vi "Stage Monitor.vi"() -> ()   [LabVIEW 2014]
uses:
  Controls/StageStates.ctl
panel:
  in  "P541 Only":bool
  in  "Monitoring":bool
  in  "Exit":bool
  out "Monitor 5":cluster{"Numeric":dbl}(graph) caption="N664"
  out "Monitor 4":cluster{"Numeric":dbl, "Numeric":dbl}(graph) caption="N664"
  out "Monitor 3":T1(graph) caption="N664"
  out "Monitor 2":T1(graph) caption="N664"
  out "Monitor 1":cluster{"Numeric":dbl}(graph) caption="N664"
  in  "Stages":T2
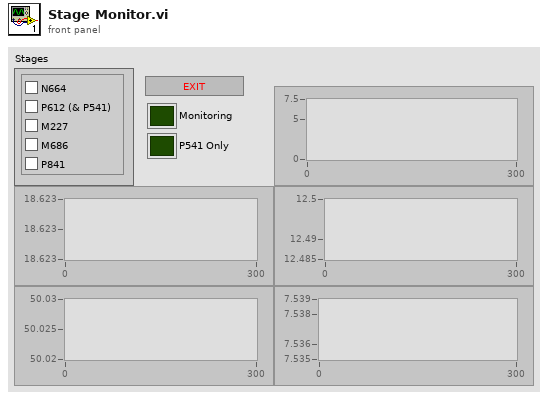
[diagram p1: front panel]
types:
  T1 = cluster{"Numeric":dbl, "Numeric":dbl, "Numeric":dbl}
  T2 = cluster{"N664":bool, "P612":bool, "M227":bool, "M686":bool, "P841":bool}
  T3 = enum8{"Enabled", "Disabled", "Disabled and Grayed Out"}
  T4 = typedef "StageStates.ctl" = enum16{"POSITION", "MVR", "MOVE", "HALT", "ONTARGET", "ERROR", "EXIT", "HOME", "ZEROPOS", "NANOPOS", "QUIT", "ANALOG"}
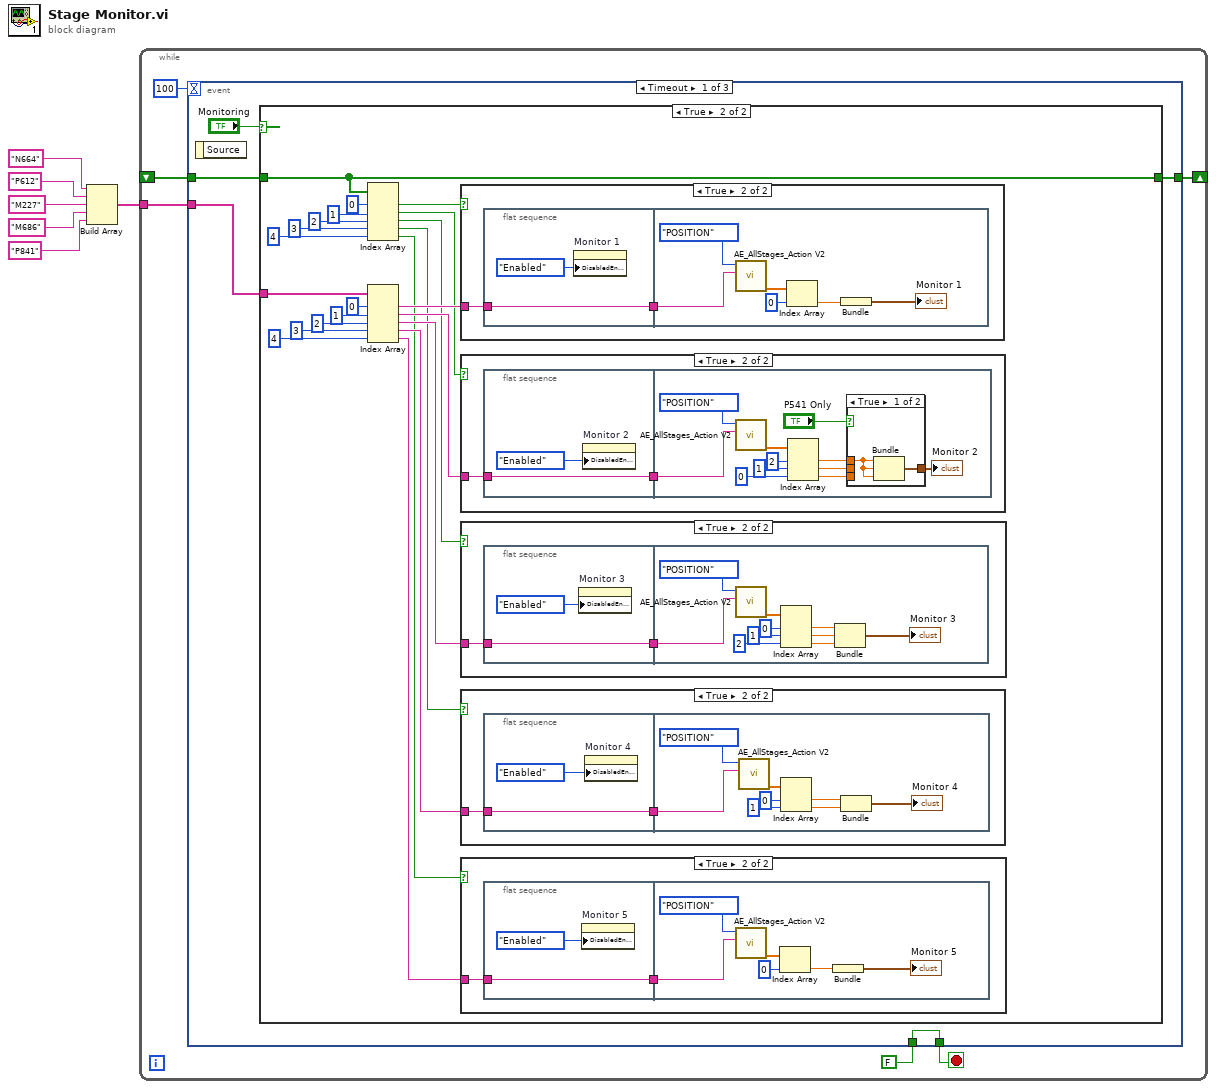
[diagram p0: block diagram]
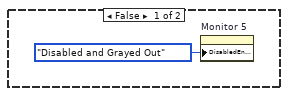
[diagram p3: hidden frame]
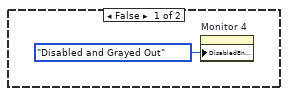
[diagram p4: hidden frame]
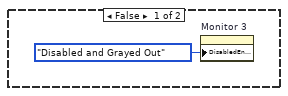
[diagram p5: hidden frame]
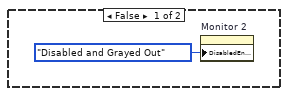
[diagram p6: hidden frame]
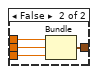
[diagram p7: hidden frame]
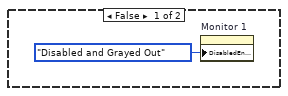
[diagram p8: hidden frame]
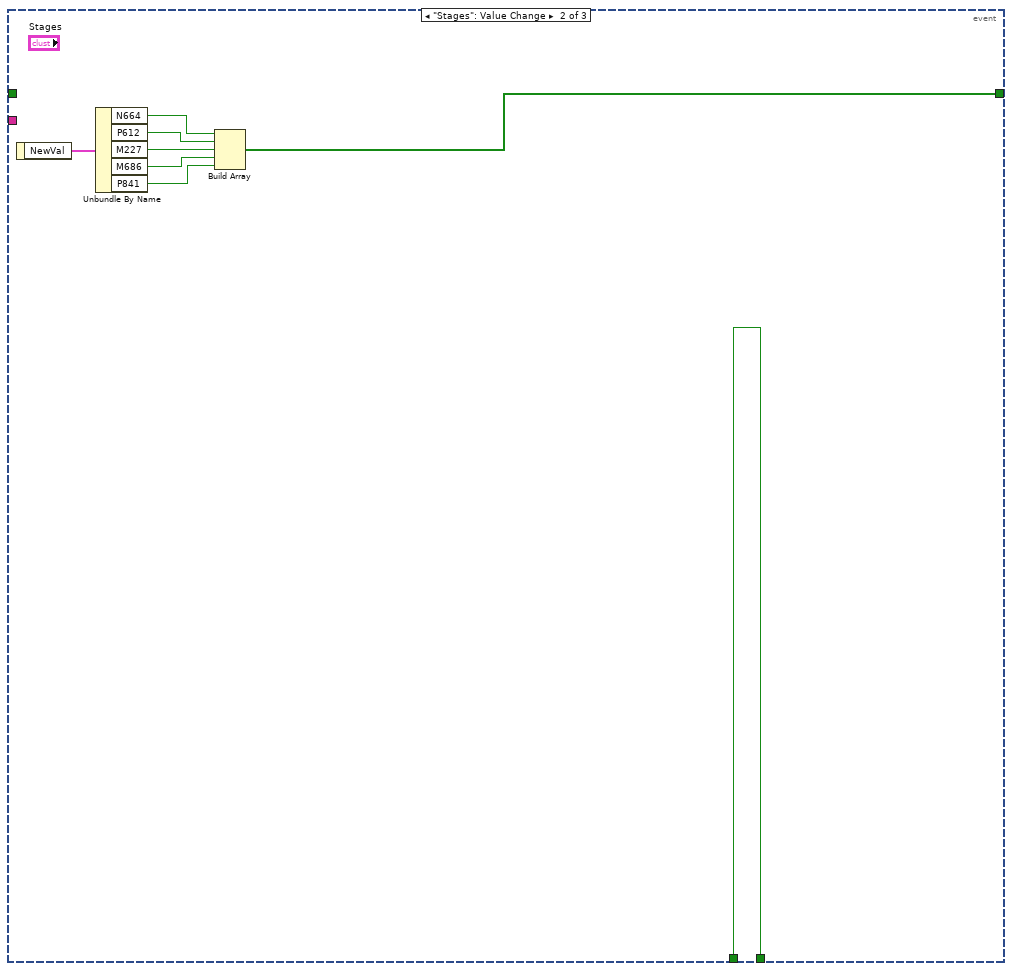
[diagram p9: hidden frame]
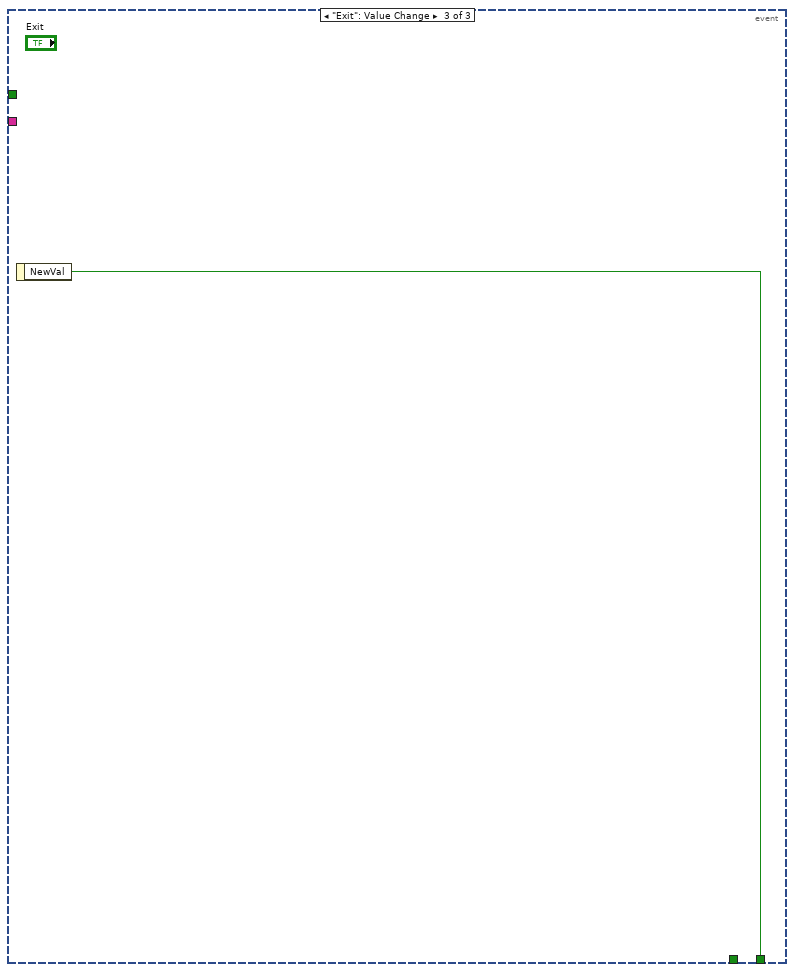
[diagram p10: hidden frame]
diagram:
  n1 = Build Array("N664", "P612", "M227", "M686", "P841") -> (w1:string[])
  n2 = while {
    shift-right: [w9] -> _
    shift-left: _ -> [w8]
    tunnel: w1 -> [w7]
    stop <- w10 stop-if-true
    n3 = event shown="[0] Timeout" {
      selector: _ -> [_ _ _]
      dyn-events: _ -> [_ _ _]
      timeout: 100 -> [_ _ _]
      tunnel: FALSE -> [w17 w120 _]
      tunnel: [w17 w120 w121] -> w10
      tunnel: [w13 w113 _] -> w9
      tunnel: w8 -> [w15 _ _]
      tunnel: w7 -> [w14 _ _]
      event Timeout {
        n4 = event-data() -> ()  [unwired: 1 in, 1 out]
        n5 = case shown="True" "Monitoring" {
          tunnel: w15 -> [w18 w40]
          tunnel: w14 -> [_ w33]
          tunnel: [w18 w40] -> w13
          frame False {
          }
          frame True {
            n6 = Index Array(array=w40, index #1=0 ("index"), index #2=1 ("index"), index #3=2 ("index"), index #4=3 ("index"), index #5=4 ("index")) -> (element #1=w34:bool, element #2=w26:bool, element #3=w24:bool, element #4=w22:bool, element #5=w20:bool)
            n7 = Index Array(array=w33, index #1=0 ("index"), index #2=1 ("index"), index #3=2 ("index"), index #4=3 ("index"), index #5=4 ("index")) -> (element #1=w27:string, element #2=w25:string, element #3=w23:string, element #4=w21:string, element #5=w19:string)
            n8 = case shown="True" w34 {
              tunnel: w27 -> [_ w103]
              frame False {
                n9 = property on="Monitor 1" class="WFChart (strict)"("DisabledEnum"=T3."Disabled and Grayed Out" ("Disabled")) -> ()  [unwired: 2 in, 2 out]
              }
              frame True {
                n10 = flat-sequence {
                  tunnel: [w105] -> w104
                  tunnel: w103 -> [w105]
                  tunnel: w104 -> [w111]
                  frame #0 {
                    n11 = property on="Monitor 1" class="WFChart (strict)"("DisabledEnum"=T3."Enabled" ("Disabled")) -> ()  [unwired: 2 in, 2 out]
                  }
                  frame #1 {
                    n12 = call "AE_AllStages_Action V2.vi"("Stage ID"=w111, "Action"=StageStates."POSITION") -> ("Position Out"=w110:dbl[])  [unwired: 7 in, 2 out]
                    n13 = Index Array(array=w110, index=0) -> (element=w108:dbl)
                    n14 = Bundle("Numeric"=w108) -> (→"Monitor 1":cluster{"Numeric":dbl})  [unwired: 1 in]
                  }
                }
              }
            }
            n15 = case shown="True" w26 {
              tunnel: w25 -> [_ w81]
              frame False {
                n16 = property on="Monitor 2" class="WFChart (strict)"("DisabledEnum"=T3."Disabled and Grayed Out" ("Disabled")) -> ()  [unwired: 2 in, 2 out]
              }
              frame True {
                n17 = flat-sequence {
                  tunnel: [w83] -> w82
                  tunnel: w81 -> [w83]
                  tunnel: w82 -> [w94]
                  frame #0 {
                    n18 = property on="Monitor 2" class="WFChart (strict)"("DisabledEnum"=T3."Enabled" ("Disabled")) -> ()  [unwired: 2 in, 2 out]
                  }
                  frame #1 {
                    n19 = call "AE_AllStages_Action V2.vi"("Stage ID"=w94, "Action"=StageStates."POSITION") -> ("Position Out"=w93:dbl[])  [unwired: 7 in, 2 out]
                    n20 = Index Array(array=w93, index #1=2 ("index"), index #2=1 ("index"), index #3=0 ("index")) -> (element #1=w89:dbl, element #2=w88:dbl, element #3=w87:dbl)
                    n21 = case shown="True" "P541 Only" {
                      tunnel: w89 -> [w97 w101]
                      tunnel: w88 -> [_ w100]
                      tunnel: w87 -> [_ w99]
                      tunnel: [w96 w98] -> w85
                      frame True {
                        n22 = Bundle("Numeric"=w97, "Numeric"=w97, "Numeric"=w97) -> (w96:T1)  [unwired: 1 in]
                      }
                      frame False {
                        n23 = Bundle("Numeric"=w101, "Numeric"=w100, "Numeric"=w99) -> (w98:T1)  [unwired: 1 in]
                      }
                    }
                    "Monitor 2" <- w85
                  }
                }
              }
            }
            n24 = case shown="True" w24 {
              tunnel: w23 -> [_ w66]
              frame False {
                n25 = property on="Monitor 3" class="WFChart (strict)"("DisabledEnum"=T3."Disabled and Grayed Out" ("Disabled")) -> ()  [unwired: 2 in, 2 out]
              }
              frame True {
                n26 = flat-sequence {
                  tunnel: [w68] -> w67
                  tunnel: w66 -> [w68]
                  tunnel: w67 -> [w78]
                  frame #0 {
                    n27 = property on="Monitor 3" class="WFChart (strict)"("DisabledEnum"=T3."Enabled" ("Disabled")) -> ()  [unwired: 2 in, 2 out]
                  }
                  frame #1 {
                    n28 = call "AE_AllStages_Action V2.vi"("Stage ID"=w78, "Action"=StageStates."POSITION") -> ("Position Out"=w77:dbl[])  [unwired: 7 in, 2 out]
                    n29 = Index Array(array=w77, index #1=0 ("index"), index #2=1 ("index"), index #3=2 ("index")) -> (element #1=w73:dbl, element #2=w72:dbl, element #3=w71:dbl)
                    n30 = Bundle("Numeric"=w73, "Numeric"=w72, "Numeric"=w71) -> (→"Monitor 3":T1)  [unwired: 1 in]
                  }
                }
              }
            }
            n31 = case shown="True" w22 {
              tunnel: w21 -> [_ w53]
              frame False {
                n32 = property on="Monitor 4" class="WFChart (strict)"("DisabledEnum"=T3."Disabled and Grayed Out" ("Disabled")) -> ()  [unwired: 2 in, 2 out]
              }
              frame True {
                n33 = flat-sequence {
                  tunnel: [w55] -> w54
                  tunnel: w53 -> [w55]
                  tunnel: w54 -> [w63]
                  frame #0 {
                    n34 = property on="Monitor 4" class="WFChart (strict)"("DisabledEnum"=T3."Enabled" ("Disabled")) -> ()  [unwired: 2 in, 2 out]
                  }
                  frame #1 {
                    n35 = call "AE_AllStages_Action V2.vi"("Stage ID"=w63, "Action"=StageStates."POSITION") -> ("Position Out"=w62:dbl[])  [unwired: 7 in, 2 out]
                    n36 = Index Array(array=w62, index #1=0 ("index"), index #2=1 ("index")) -> (element #1=w59:dbl, element #2=w58:dbl)
                    n37 = Bundle("Numeric"=w59, "Numeric"=w58) -> (→"Monitor 4":cluster{"Numeric":dbl, "Numeric":dbl})  [unwired: 1 in]
                  }
                }
              }
            }
            n38 = case shown="True" w20 {
              tunnel: w19 -> [_ w42]
              frame False {
                n39 = property on="Monitor 5" class="WFChart (strict)"("DisabledEnum"=T3."Disabled and Grayed Out" ("Disabled")) -> ()  [unwired: 2 in, 2 out]
              }
              frame True {
                n40 = flat-sequence {
                  tunnel: [w44] -> w43
                  tunnel: w42 -> [w44]
                  tunnel: w43 -> [w50]
                  frame #0 {
                    n41 = property on="Monitor 5" class="WFChart (strict)"("DisabledEnum"=T3."Enabled" ("Disabled")) -> ()  [unwired: 2 in, 2 out]
                  }
                  frame #1 {
                    n42 = call "AE_AllStages_Action V2.vi"("Stage ID"=w50, "Action"=StageStates."POSITION") -> ("Position Out"=w49:dbl[])  [unwired: 7 in, 2 out]
                    n43 = Index Array(array=w49, index=0) -> (element=w47:dbl)
                    n44 = Bundle("Numeric"=w47) -> (→"Monitor 5":cluster{"Numeric":dbl})  [unwired: 1 in]
                  }
                }
              }
            }
          }
        }
      }
      event "Stages": Value Change {
        n45 = event-data() -> ("NewVal"=w114:T2)  [unwired: 1 in]
        n46 = Unbundle By Name(w114) -> ("N664"=w119:bool, "P612"=w118:bool, "M227"=w117:bool, "M686"=w116:bool, "P841"=w115:bool)
        n47 = Build Array(w119, w118, w117, w116, w115) -> (w113:bool[])
      }
      event "Exit": Value Change {
        n48 = event-data() -> ("NewVal"=w121:bool)  [unwired: 1 in]
      }
    }
  }
